vi "AddNestedEnqueuer.vi"(8 "error in (no error)":errorcluster, 10 "Nested Actor's Enqueuer":refnum<class "Message Enqueuer.lvclass">, 11 "ServiceManager-Comms in":refnum<class "ServiceManager-Comms.lvclass">) -> (0 "error out":errorcluster, 3 "ServiceManager-Comms out":refnum<class "ServiceManager-Comms.lvclass">)   [LabVIEW 2020, in "ServiceManager-Comms.lvlib" / "ServiceManager-Comms.lvclass"]
uses:
  ServiceManager-Comms.lvclass
  <vilib>/ActorFramework/Message Enqueuer/Message Enqueuer.lvclass
  ServiceManager-Comms.lvclass/ServiceManager-Comms.ctl
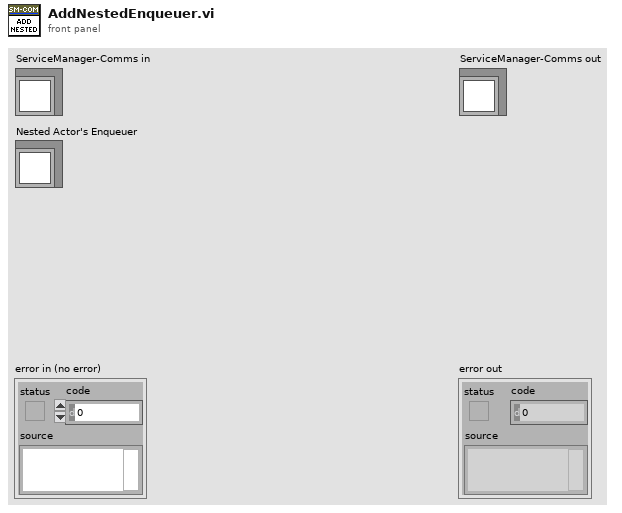
[diagram p1: front panel]
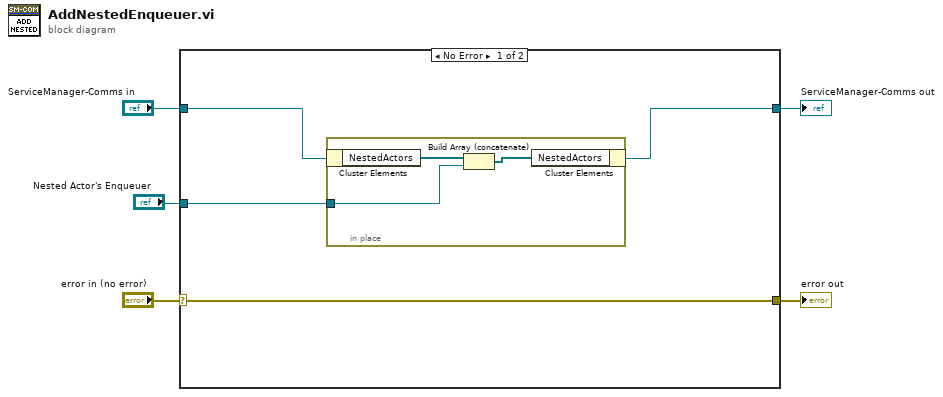
[diagram p0: block diagram]
diagram:
  n1 = case shown="No Error" "error in (no error)" {
    selector: "error in (no error)" -> [w9 w14]
    tunnel: [w9 w14] -> w4
    tunnel: [w6 w13] -> w2
    tunnel: "ServiceManager-Comms in" -> [w8 w13]
    tunnel: "Nested Actor's Enqueuer" -> [w7 _]
    frame No Error {
      n2 = in-place {
        in-place-border: w7 -> [w10]
        n3 = in-place-cluster #1(w8) -> ("NestedActors"=w12:refnum<class "Message Enqueuer.lvclass">[])
        n4 = Build Array (concatenate)(w12, w10) -> (w11:refnum<class "Message Enqueuer.lvclass">[])
        n5 = in-place-cluster #1("NestedActors"=w11) -> (w6:refnum<class "ServiceManager-Comms.lvclass">)
      }
    }
    frame Error {
    }
  }
  "error out" <- w4
  "ServiceManager-Comms out" <- w2
